vi "niDTS BT INSTR RX Configure PortMapping.vi"(8 "error in (no error)":errorcluster, 11 "niDTS BT INSTR RX in":refnum<class "niDTS BT INSTR RX.lvclass">) -> (0 "error out":errorcluster, 3 "niDTS BT INSTR RX out":refnum<class "niDTS BT INSTR RX.lvclass">)   [LabVIEW 2015, in "niDTS BT.lvlib" / "niDTS BT INSTR RX.lvclass"]
uses:
  niDTS BT INSTR RX.lvclass
  niDTS BT INSTR RX.lvclass/niDTS BT INSTR RX.ctl
  RiviInstDriver/niRfsgBT/Objects/niRfsgBt.lvclass
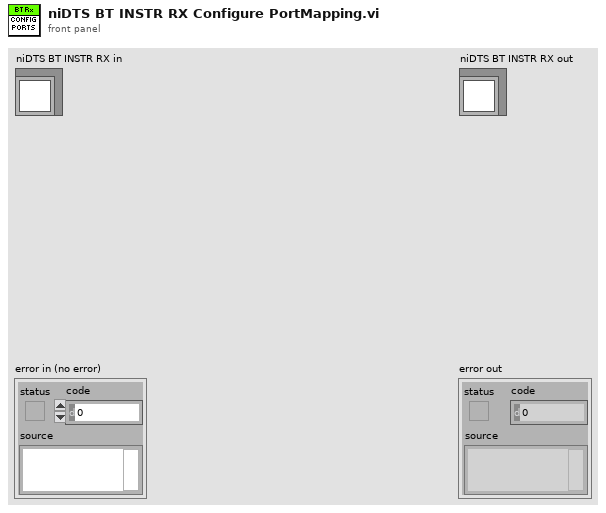
[diagram p1: front panel]
types:
  T1 = typedef "niRfsgBT.lvclass/niRfsgBT INC Handle.ctl" = refnum<data-value>
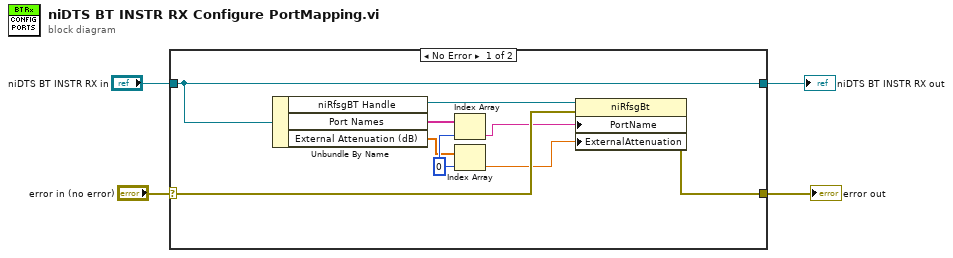
[diagram p0: block diagram]
diagram:
  n1 = case shown="No Error" "error in (no error)" {
    selector: "error in (no error)" -> [w11 w15]
    tunnel: [w10 w15] -> w3
    tunnel: [w13 w14] -> w1
    tunnel: "niDTS BT INSTR RX in" -> [w13 w14]
    frame No Error {
      w8 = 0 ("index")
      n2 = Unbundle By Name(w13) -> ("niRfsgBT Handle"=w12:T1, "Port Names"=w9:string[], "External Attenuation (dB)"=w6:dbl[])
      n3 = Index Array(array=w9, index=w8) -> (element=w7:string)
      n4 = Index Array(array=w6, index=w8) -> (element=w5:dbl)
      n5 = property class="niRfsgBt"(reference=w12, error in=w11, "PortName"=w7, "ExternalAttenuation"=w5) -> (error out=w10:errorcluster)  [unwired: 1 out]
    }
    frame Error {
    }
  }
  "error out" <- w3
  "niDTS BT INSTR RX out" <- w1
